vi "CreateCreepSamples.vi"(0 "t0":dbl, 5 "input cluster":T1, 7 "outputLength":i32, 9 "loadInNewtons":dbl, 11 "rampTimeInSeconds":dbl) -> (8 "output array":dbl[][](array[numeric]))   [LabVIEW 2009]
uses:
  samplePlaybackGenerator.dll
panel:
  out "Number of points":i32=1000
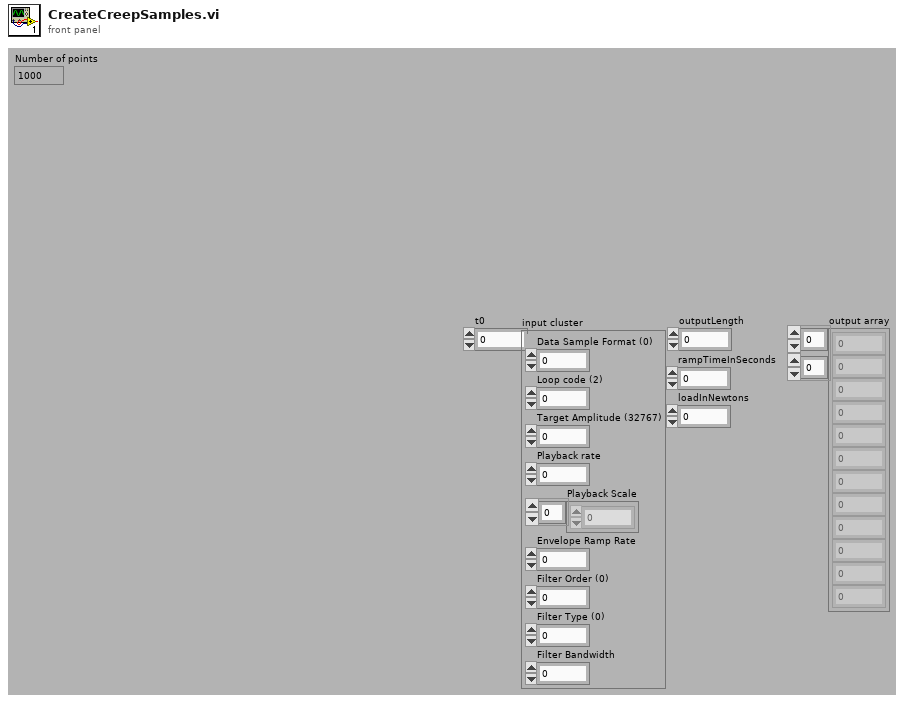
[diagram p1: front panel]
types:
  T1 = cluster{"Data Sample Format (0)":i8, "Loop code (2)":i8, "Target Amplitude (32767)":i16, "Playback rate":dbl, "Playback Scale":dbl[], "Envelope Ramp Rate":dbl, "Filter Order (0)":i8, "Filter Type (0)":i8, "Filter Bandwidth":dbl}
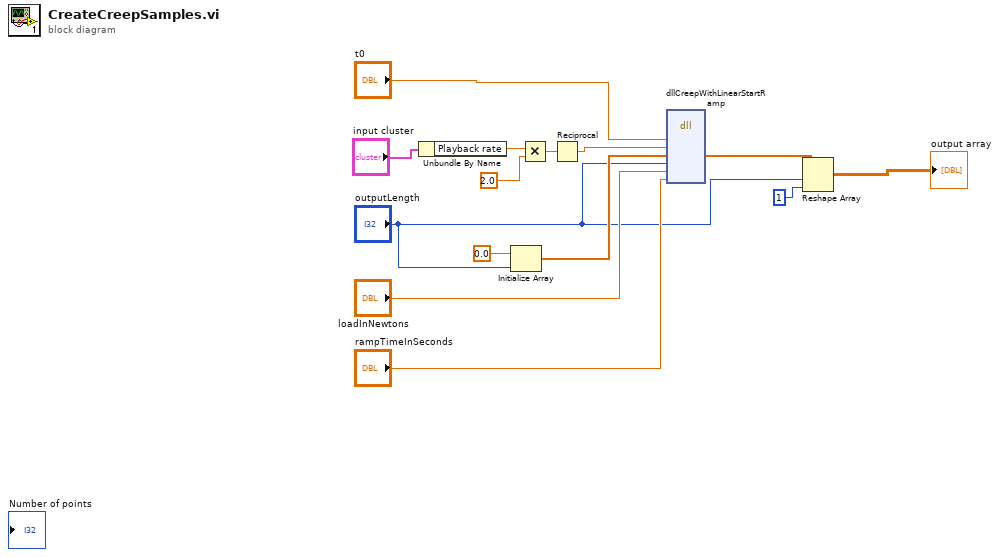
[diagram p0: block diagram]
diagram:
  n1 = Unbundle By Name("input cluster") -> ("Playback rate"=w2:dbl)
  n2 = Initialize Array(0.0 ("element"), "outputLength") -> (w12:dbl[])
  n3 = Multiply(x=w2, y=2.0) -> (x*y=w3:dbl)
  n4 = Reciprocal(x=w3) -> (1/x=w13:dbl)
  n5 = dll-call lib="C:/instronLabviewPrograms/csm_setpoint_and_ramp_lumikki/lib/samplePlaybackGenerator.dll" fn="dllCreepWithLinearStartRamp"("t0"="t0", "tStep"=w13, "output"=w12, "outputLength"="outputLength", "loadInNewtons"="loadInNewtons", "rampTimeInSeconds"="rampTimeInSeconds") -> ("output"=w11:dbl[])  [unwired: 9 in, 2 out]
  n6 = Reshape Array(w11, "outputLength", 1 ("dimension size")) -> (→"output array":dbl[][])
